vi "Read Warning_.vi"(8 "error in (no error)":errorcluster, 11 "AssertError in":refnum<class "AssertError.lvclass">) -> (0 "error out":errorcluster, 2 "Warning?":bool, 3 "AssertError out":refnum<class "AssertError.lvclass">)   [LabVIEW 2021, in "Bananas.lvlib" / "AssertError.lvclass"]
uses:
  AssertError.lvclass
  AssertError.lvclass/AssertError.ctl
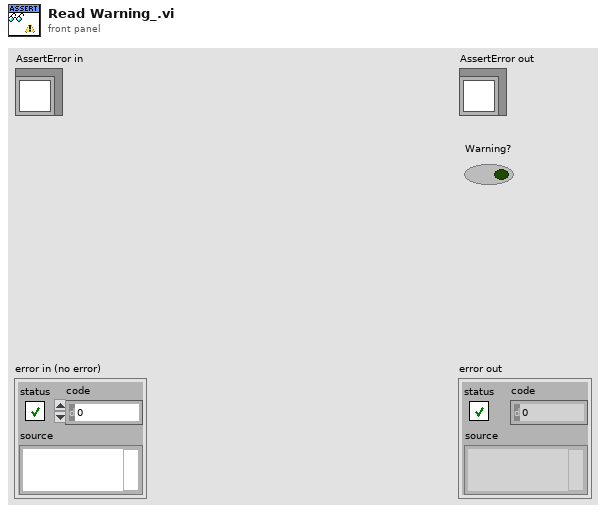
[diagram p1: front panel]
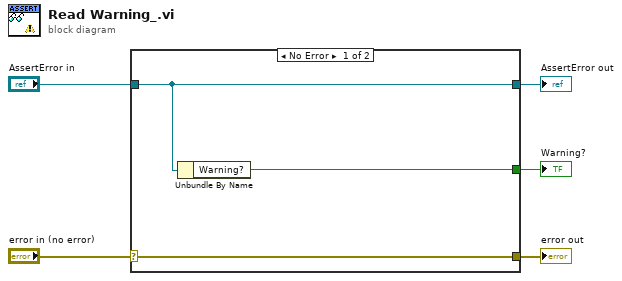
[diagram p0: block diagram]
diagram:
  n1 = case shown="No Error" "error in (no error)" {
    selector: "error in (no error)" -> [w8 w9]
    tunnel: [w8 w9] -> w4
    tunnel: [w7 w10] -> w2
    tunnel: "AssertError in" -> [w7 w10]
    tunnel: [w6 _] -> w1
    frame No Error {
      n2 = Unbundle By Name(w7) -> ("Warning?"=w6:bool)
    }
    frame Error {
    }
  }
  "error out" <- w4
  "AssertError out" <- w2
  "Warning?" <- w1
